vi "Read Set.vi"(0 "VISA resource name":refnum<visa-resource-name>, 11 "error in (no error)":errorcluster) -> (1 "Local Lockout":u32(ring) items=["Off", "On"], 2 "ATTN":u32(ring) items=["Off", "On"], 3 "Run/Stop":u32(ring)=1 items=["Stop", "Run"], 4 "VISA resource name out":refnum<visa-resource-name>, 5 "Wavelength (nnnn)":dbl[unit], 6 "AVG":u32(ring) items=["Slow", "Medium", "Fast"], 9 "Range (1:8)":u32(ring) items=["Auto", "Lowest", "2", "3", "4", "5", "6", "7", "Highest"], 10 "Units":u32(ring)=1 items=["W"=1, "dB"=2, "dBm"=3, "REL"=4], 12 "Backlight":u32(ring) items=["Off", "Low", "High"], 13 "Beeper":u32(ring) items=["Off", "On"], 14 "Zero":u32(ring) items=["Off", "On"], 15 "error out":errorcluster)   [LabVIEW 2009]
doc: "Reads 1830-C options in succession and outputs their values.\n\nNote: Cannot tell if AutoRange is active."
uses:
  Newport 1830-C/Newport 1830-C.lvlib
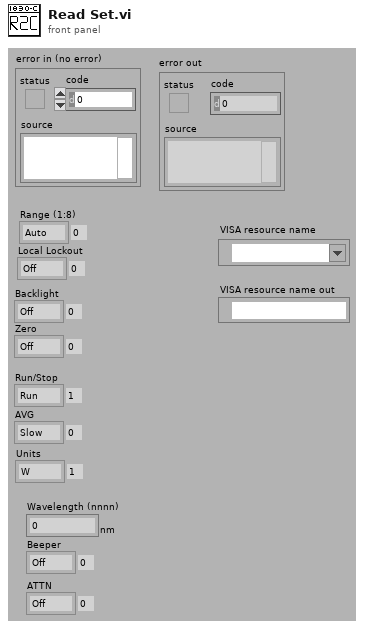
[diagram p1: front panel]
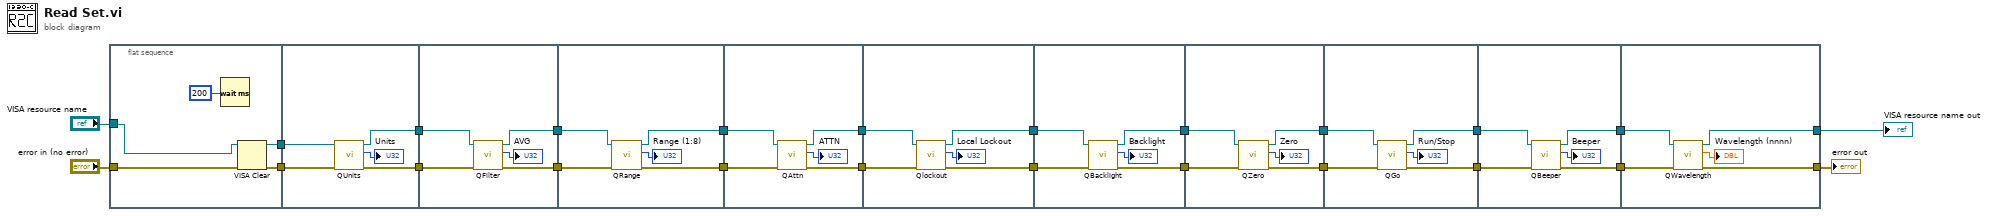
[diagram p0: block diagram]
diagram:
  n1 = flat-sequence {
    tunnel: [w29] -> w4
    tunnel: [w28] -> w3
    tunnel: "VISA resource name" -> [w26]
    tunnel: "error in (no error)" -> [w27]
    tunnel: [w34] -> w24
    tunnel: [w31] -> w14
    tunnel: w4 -> [w33]
    tunnel: w3 -> [w32]
    tunnel: w24 -> [w39]
    tunnel: [w38] -> w23
    tunnel: w14 -> [w37]
    tunnel: [w36] -> w13
    tunnel: w23 -> [w44]
    tunnel: [w43] -> w22
    tunnel: w13 -> [w42]
    tunnel: [w41] -> w12
    tunnel: w22 -> [w49]
    tunnel: [w48] -> w21
    tunnel: w12 -> [w47]
    tunnel: [w46] -> w11
    tunnel: w21 -> [w54]
    tunnel: [w53] -> w20
    tunnel: w11 -> [w52]
    tunnel: [w51] -> w10
    tunnel: w20 -> [w59]
    tunnel: [w58] -> w19
    tunnel: w10 -> [w57]
    tunnel: [w56] -> w9
    tunnel: w19 -> [w64]
    tunnel: [w63] -> w18
    tunnel: w9 -> [w62]
    tunnel: [w61] -> w8
    tunnel: w18 -> [w69]
    tunnel: [w68] -> w17
    tunnel: w8 -> [w67]
    tunnel: [w66] -> w7
    tunnel: w17 -> [w74]
    tunnel: [w73] -> w16
    tunnel: w7 -> [w72]
    tunnel: [w71] -> w6
    tunnel: w16 -> [w79]
    tunnel: [w78] -> w15
    tunnel: w6 -> [w77]
    tunnel: [w76] -> w5
    frame #0 {
      n2 = Wait (ms)(milliseconds to wait=u32 200) -> ()  [unwired: 1 out]
      n3 = VISA Clear(VISA resource name=w26, error in (no error)=w27) -> (VISA resource name out=w29:refnum<visa-resource-name>, error out=w28:errorcluster)
    }
    frame #1 {
      n4 = call "QUnits.vi"("error in (no error)"=w32, "VISA resource name"=w33) -> ("error out"=w31:errorcluster, "Units"=→"Units":u32, "VISA resource name out"=w34:refnum<visa-resource-name>)  [unwired: 6 in, 1 out]
    }
    frame #2 {
      n5 = call "QFilter.vi"("error in (no error)"=w37, "VISA resource name"=w39) -> ("error out"=w36:errorcluster, "Filter State"=→"AVG":u32, "VISA resource name out"=w38:refnum<visa-resource-name>)  [unwired: 7 in]
    }
    frame #3 {
      n6 = call "QRange.vi"("error in (no error)"=w42, "VISA resource name"=w44) -> ("error out"=w41:errorcluster, "Range"=→"Range (1:8)":u32, "VISA resource name out"=w43:refnum<visa-resource-name>)  [unwired: 7 in]
    }
    frame #4 {
      n7 = call "QAttn.vi"("error in (no error)"=w47, "VISA resource name"=w49) -> ("error out"=w46:errorcluster, "Attn State"=→"ATTN":u32, "VISA resource name out"=w48:refnum<visa-resource-name>)  [unwired: 7 in]
    }
    frame #5 {
      n8 = call "Qlockout.vi"("error in (no error)"=w52, "VISA resource name"=w54) -> ("error out"=w51:errorcluster, "Lockout State"=→"Local Lockout":u32, "VISA resource name out"=w53:refnum<visa-resource-name>)  [unwired: 7 in]
    }
    frame #6 {
      n9 = call "QBacklight.vi"("error in (no error)"=w57, "VISA resource name"=w59) -> ("error out"=w56:errorcluster, "BKLT State"=→"Backlight":u32, "VISA resource name out"=w58:refnum<visa-resource-name>)  [unwired: 7 in]
    }
    frame #7 {
      n10 = call "QZero.vi"("error in (no error)"=w62, "VISA resource name"=w64) -> ("error out"=w61:errorcluster, "Zero State"=→"Zero":u32, "VISA resource name out"=w63:refnum<visa-resource-name>)  [unwired: 7 in]
    }
    frame #8 {
      n11 = call "QGo.vi"("error in (no error)"=w67, "VISA resource name"=w69) -> ("error out"=w66:errorcluster, "Go State"=→"Run/Stop":u32, "VISA resource name out"=w68:refnum<visa-resource-name>)  [unwired: 7 in]
    }
    frame #9 {
      n12 = call "QBeeper.vi"("error in (no error)"=w72, "VISA resource name"=w74) -> ("error out"=w71:errorcluster, "Beeper State"=→"Beeper":u32, "VISA resource name out"=w73:refnum<visa-resource-name>)  [unwired: 7 in]
    }
    frame #10 {
      n13 = call "QWavelength.vi"("error in (no error)"=w77, "VISA resource name"=w79) -> ("error out"=w76:errorcluster, "Wavelength"=→"Wavelength (nnnn)":dbl[unit], "VISA resource name out"=w78:refnum<visa-resource-name>)  [unwired: 7 in]
    }
  }
  "error out" <- w5
  "VISA resource name out" <- w15
